vi "Read Proto Test Configuration.vi"(8 "error in (no error)":errorcluster, 11 "Protocol Verification Test in":refnum<class "Protocol Verification Test.lvclass">) -> (0 "error out":errorcluster, 2 "Cluster":T1, 3 "Protocol Verification Test out":refnum<class "Protocol Verification Test.lvclass">)   [LabVIEW 2017, in "Protocol Verification Test.lvlib" / "Protocol Verification Test.lvclass"]
uses:
  Protocol Verification Test.lvclass
  Protocol Verification Configuration.ctl
  Protocol Verification Test.lvclass/Protocol Verification Test.ctl
  Protocol Verification Test.lvlib
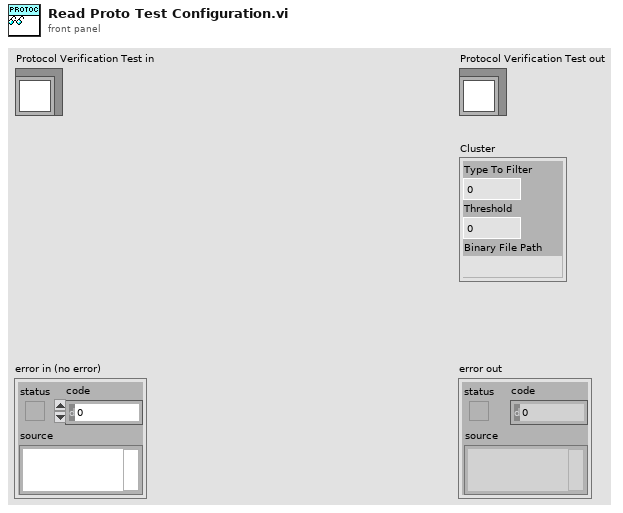
[diagram p1: front panel]
types:
  T1 = typedef "Protocol Verification Test.lvlib/Protocol Verification Configuration.ctl" = cluster{"Type To Filter":i32, "Threshold":dbl, "Binary File Path":path}
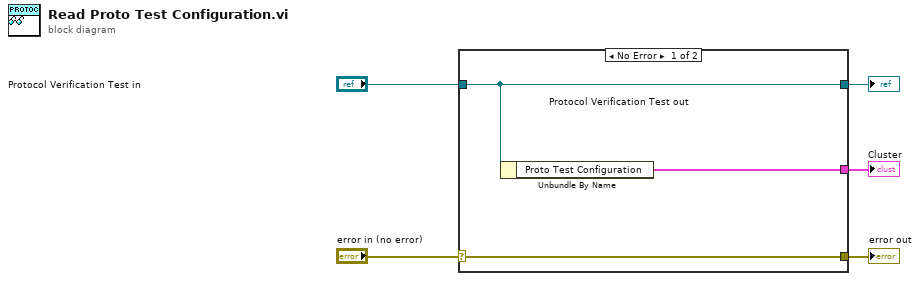
[diagram p0: block diagram]
diagram:
  n1 = case shown="No Error" "error in (no error)" {
    selector: "error in (no error)" -> [w8 w9]
    tunnel: [w8 w9] -> w4
    tunnel: [w7 w10] -> w2
    tunnel: "Protocol Verification Test in" -> [w7 w10]
    tunnel: [w6 _] -> w1
    frame No Error {
      n2 = Unbundle By Name(w7) -> ("Proto Test Configuration"=w6:T1)
    }
    frame Error {
    }
  }
  "error out" <- w4
  "Protocol Verification Test out" <- w2
  "Cluster" <- w1
